vi "AlliGator Load HDF5 FLI Dataset Information.vi"(8 "Error In":errorcluster, 11 "File Path":path) -> (0 "error out":errorcluster, 1 "Data Description":string, 2 "Metadata":string, 3 "FLI Data File Information":T1, 4 "elapsed (relative) seconds":dbl)   [LabVIEW 2021, in "AlliGator HDF5.lvlib"]
doc: "Loads HDF5 FLI dataset information."
uses:
  AlliGator HDF5.lvlib
  AlliGator FLI Data File Information.ctl
  Phasor/Phasor Fluorescence Lifetime Parameters v3.ctl
  AlliGator FLI Dataset Type.ctl
  AlliGator HDF5 FLI File Loading Information v0.2.ctl
  Phasor/Fluorescence Lifetime Parameters.ctl
  AlliGator HDF5 FLI File Loading Information v0.6.ctl
  SwissSPAD/SwissSPAD Live_Image ROI Information.ctl
  AlliGator Image Binning Options.ctl
  Phasor/Phasor Fluorescence Lifetime Parameters v2.ctl
  <vilib>/addons/h5labview2/base/lib_path.vi
  <vilib>/addons/h5labview2/base/H5Equery.vi
  <vilib>/Utility/error.llb/Error Cluster From Error Code.vi
  AlliGator Load Single HDF5 Gate Image v 0.2b.vi
  AlliGator Load Single HDF5 Gate Image v 0.3b.vi
  AlliGator Load Single Gate Image from HDF5 v 0.6b.vi
  <vilib>/addons/h5labview2/base/hid_t.ctl
  <vilib>/addons/h5labview2/dataset/H5Dread.llb/H5Dread.xnode
  <vilib>/ErrorRing/Error Ring.xnode
  <vilib>/addons/h5labview2/file/H5F.lvlib
  <vilib>/addons/h5labview2/group/H5G.lvlib
  Time/Time.lvlib
  Phasor/Phasor.lvlib
  SwissSPAD/SwissSPAD Live.lvlib
  AlliGator Source Image.lvlib
  AlliGator Files.lvlib
  Variant/Variant.lvlib
panel:
  # "see the AlliGator License on the block diagram (Ctrl+E or Window:Show Block Diagram)"
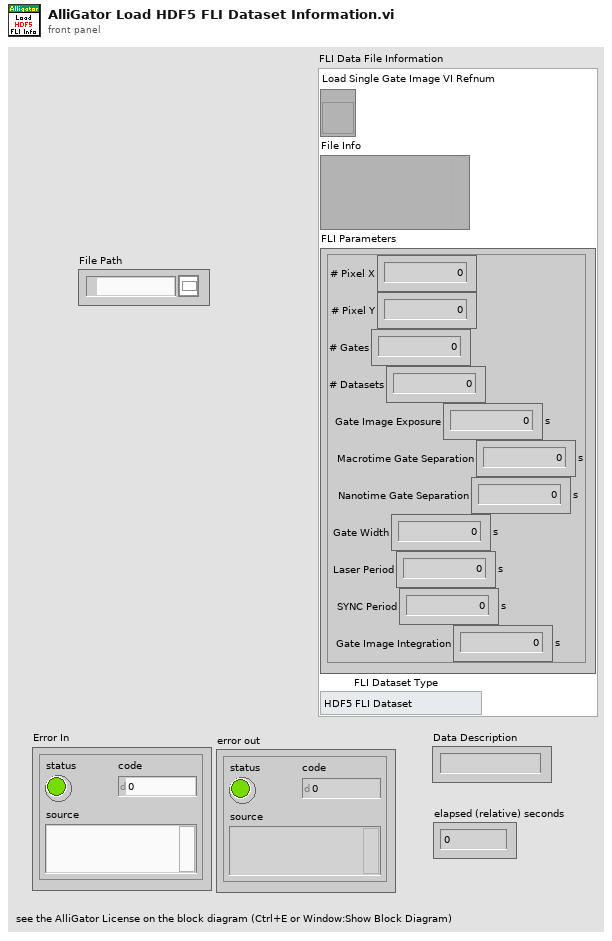
[diagram p1: front panel]
types:
  T1 = typedef "AlliGator HDF5.lvlib/AlliGator FLI Data File Information.ctl" = cluster{"Load Single Gate Image VI Refnum":refnum<vi>, "File Info":variant, "FLI Parameters":T2, "FLI Dataset Type":T3}
  T2 = typedef "Phasor.lvlib/Phasor Fluorescence Lifetime Parameters v3.ctl" = cluster{"# Pixel X":i32, "# Pixel Y":i32, "# Gates":i32, "# Datasets":i32, "Gate Image Exposure":dbl[unit], "Macrotime Gate Separation":dbl[unit], "Nanotime Gate Separation":dbl[unit], "Gate Width":dbl[unit], "Laser Period":dbl[unit], "SYNC Period":dbl[unit], "Gate Image Integration":dbl[unit]}
  T3 = typedef "AlliGator Files.lvlib/AlliGator FLI Dataset Type.ctl" = enum16{"HDF5 FLI Dataset", "Gate Image Folder", ".sdt FLI Dataset (Becker & Hickl)", ".ptu FLI Dataset (PicoQuant)", "SS1 FLI Dataset", "SS2 FLI Dataset", "I/m/phi Dataset", ".bin FLI Dataset (PicoQuant Binned)", ".bin FLI Dataset (Piccolo Binned)"}
  T4 = typedef "Phasor.lvlib/Fluorescence Lifetime Parameters.ctl" = cluster{"# Pixel X":i32, "# Pixel Y":i32, "# Gates":i32, "# Datasets":i32, "Exposure/Gate":dbl[unit], "Macrotime Gate Separation":dbl[unit], "Nanotime Gate Separation":dbl[unit], "Gate Duration":dbl[unit], "Laser Period":dbl[unit]}
  T5 = typedef "AlliGator HDF5.lvlib/AlliGator HDF5 FLI File Loading Information v0.2.ctl" = cluster{"HDF5 File Path":path}
  T6 = typedef "AlliGator HDF5.lvlib/AlliGator HDF5 FLI File Loading Information v0.6.ctl" = cluster{"HDF5 File Path":path, "Data Type":string, "# Datasets in Series":i32, "Dataset ID in Series":i32, "Channel Names":string[]}
  T7 = typedef "AlliGator Source Image.lvlib/AlliGator Image Binning Options.ctl" = cluster{"Use Image Binning":bool, "X Bin":i32, "Y Bin":i32}
  T8 = typedef "SwissSPAD Live.lvlib/SwissSPAD Live_Image ROI Information.ctl" = cluster{"Save ROI Only":bool, "Left":u16, "Top":u16, "Right":u16, "Bottom":u16, "Use Current ROI":bool}
  T9 = typedef "Phasor.lvlib/Phasor Fluorescence Lifetime Parameters v2.ctl" = cluster{"# Pixel X":i32, "# Pixel Y":i32, "# Gates":i32, "# Datasets":i32, "Exposure/Gate":dbl[unit], "Macrotime Gate Separation":dbl[unit], "Nanotime Gate Separation":dbl[unit], "Gate Duration":dbl[unit], "Laser Period":dbl[unit], "SYNC Period":dbl[unit]}
  T10 = typedef "hid_t.ctl" = i64
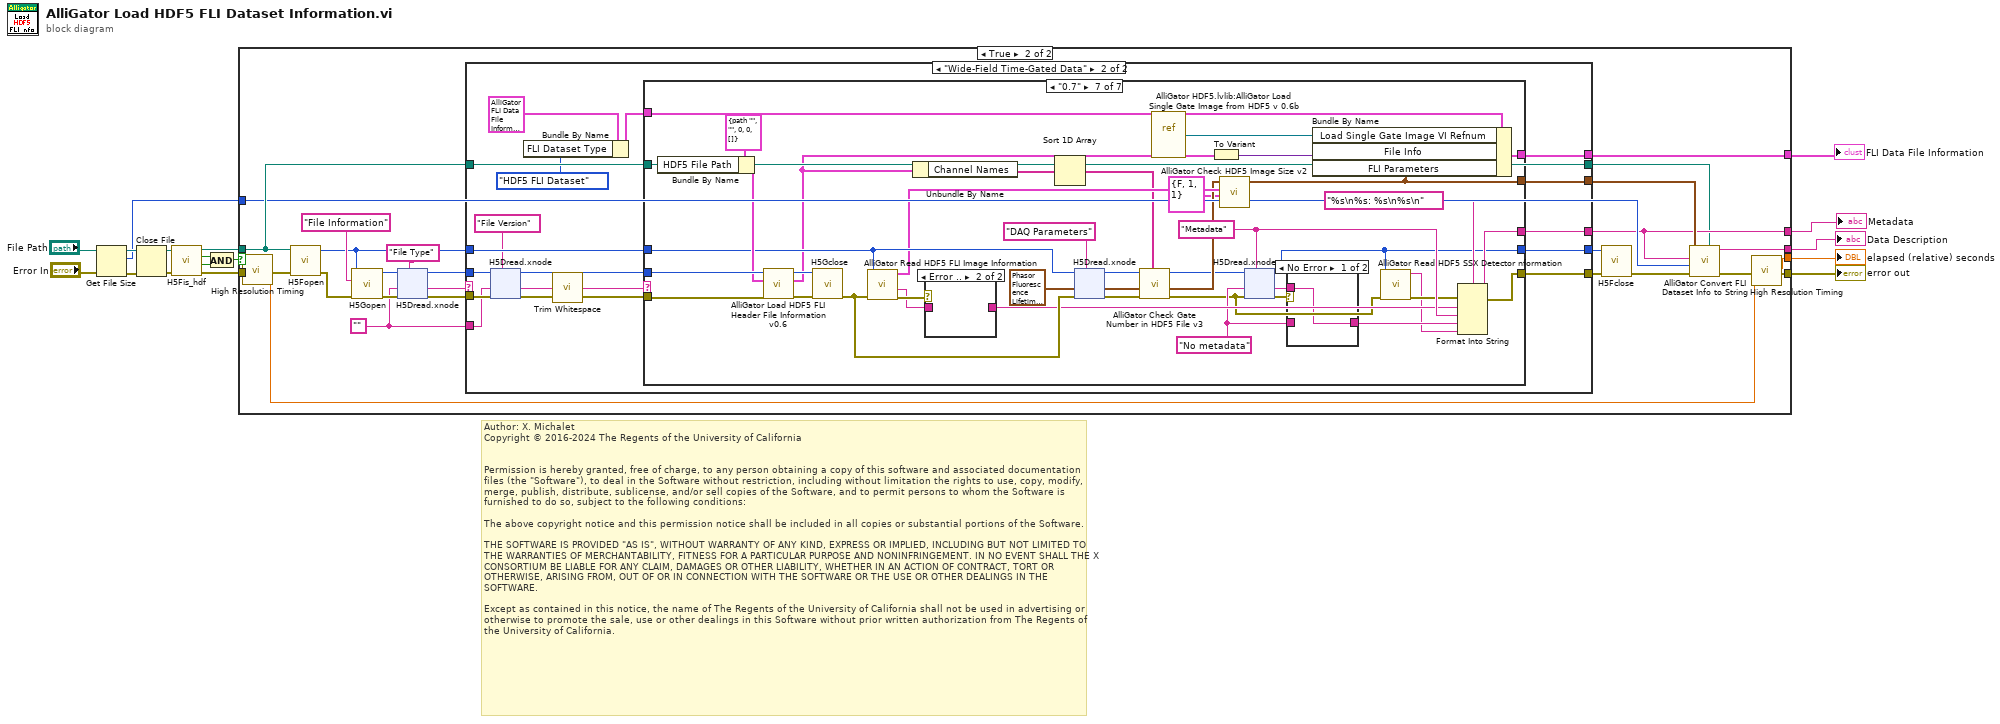
[diagram p0: block diagram]
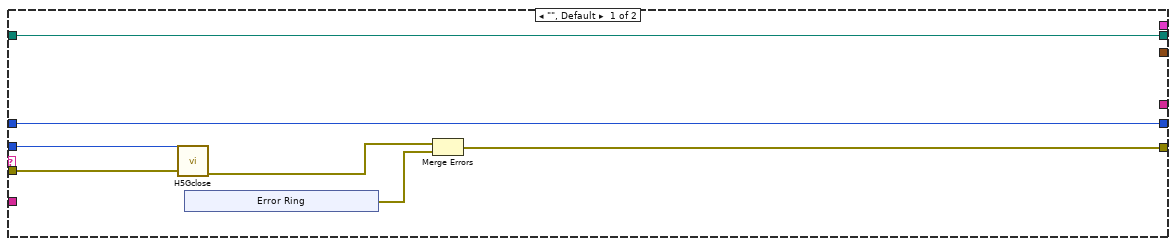
[diagram p3: hidden frame]
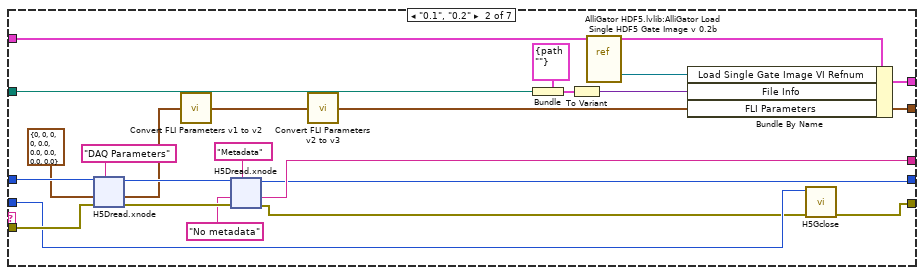
[diagram p5: hidden frame]
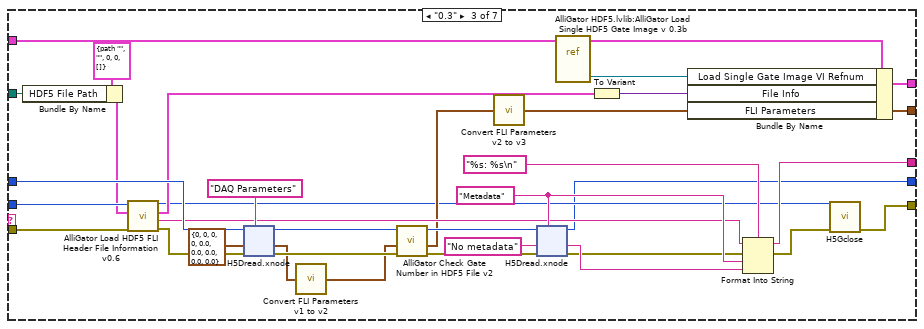
[diagram p6: hidden frame]
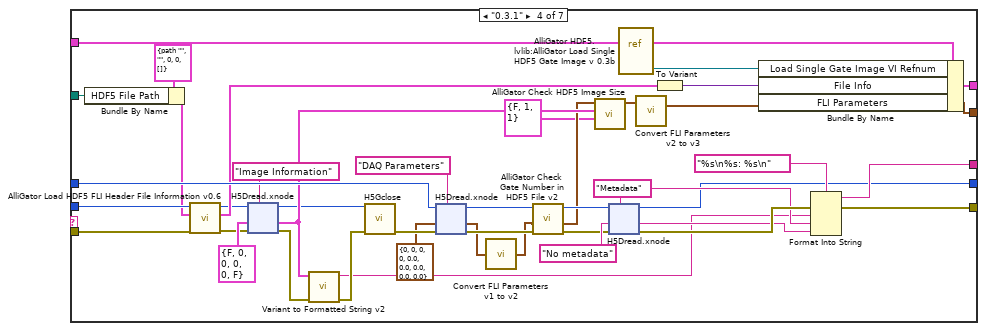
[diagram p7: hidden frame]
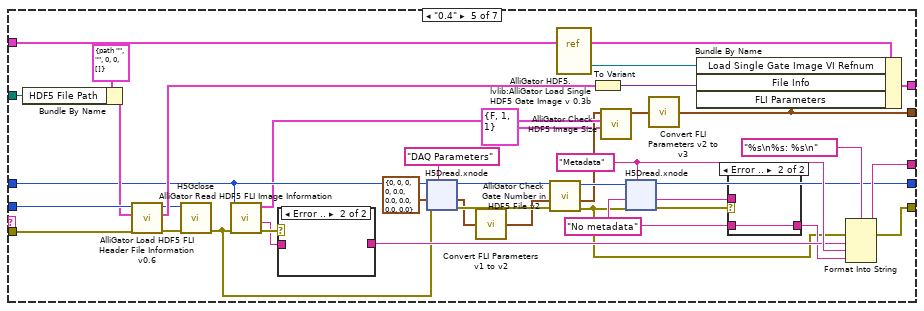
[diagram p8: hidden frame]
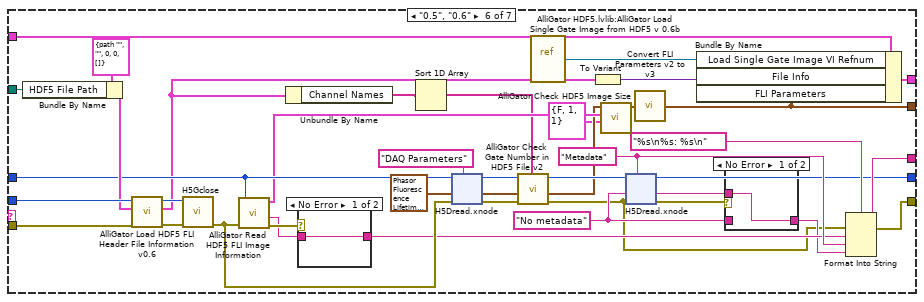
[diagram p11: hidden frame]
diagram:
  # "Author: X. Michalet\nCopyright © 2016-2024 The Regents of the University of California\n \n\nPermission is hereby granted, free of charge, to any person obtaining a copy of this software and associated documentation files (the \"Software\"), to deal in the Software without restriction, including without limitation the rights to use, copy, modify, merge, publish, distribute, sublicense, and/or sell copies of the Software, and to permit persons to whom the Software is furnished to do so, subject to the following conditions:\n\nThe above copyright notice and this permission notice shall be included in all copies or substantial portions of the Software.\n\nTHE SOFTWARE IS PROVIDED \"AS IS\", WITHOUT WARRANTY OF ANY KIND, EXPRESS OR IMPLIED, INCLUDING BUT NOT LIMITED TO THE WARRANTIES OF MERCHANTABILITY, FITNESS FOR A PARTICULAR PURPOSE AND NONINFRINGEMENT. IN NO EVENT SHALL THE X CONSORTIUM BE LIABLE FOR ANY CLAIM, DAMAGES OR OTHER LIABILITY, WHETHER IN AN ACTION OF CONTRACT, TORT OR OTHERWISE, ARISING FROM, OUT OF OR IN CONNECTION WITH THE SOFTWARE OR THE USE OR OTHER DEALINGS IN THE SOFTWARE.\n\nExcept as contained in this notice, the name of The Regents of the University of California shall not be used in advertising or otherwise to promote the sale, use or other dealings in this Software without prior written authorization from The Regents of the University of California."
  n1 = Get File Size(file="File Path", error in="Error In") -> (refnum out=w8:refnum<file>, size (in bytes)=w2:i64, 0:w9:errorcluster)
  n2 = Close File(refnum=w8, error in=w9) -> (path=w7:path, error out=w6:errorcluster)
  n3 = call <vilib>:"H5Fis_hdf.vi"("error in (no error)"=w6, "path in"=w7) -> ("error out"=w13:errorcluster, "valid?"=w16:bool, "exists?"=w17:bool, "path out"=w14:path)  [unwired: 6 in]
  n4 = And(x=w17, y=w16) -> (x .and. y?=w15:bool)
  n5 = case shown="True" w15 {
    tunnel: w14 -> [_ w27]
    tunnel: w13 -> [w18 w44]
    tunnel: [w18 w39] -> w12
    tunnel: [_ w37] -> w5
    tunnel: [_ w21] -> w4
    tunnel: [_ w26] -> w3
    tunnel: w2 -> [_ w23]
    tunnel: [_ w20] -> w1
    frame False {
    }
    frame True {
      w28 = ""
      n6 = call "High Resolution Timing.vi"("Error In"=w44) -> ("elapsed (relative) seconds"=w38:dbl, "Error Out"=w40:errorcluster)  [unwired: 16 in, 1 out]
      n7 = call <vilib>:"H5Fopen.vi"("error in (no error)"=w40, "path"=w27) -> ("error out"=w36:errorcluster, "ref out"=w31:T10)  [unwired: 8 in]
      n8 = call <vilib>:"H5Gopen.vi"("error in (no error)"=w36, "name"="File Information" ("dataset name (this)"), "ref in"=w31) -> ("error out"=w34:errorcluster, "group out"=w33:T10)  [unwired: 7 in]
      n9 = xnode "H5Dread.xnode"("dataset name (this)"="File Type", "error in (no error)"=w34, "default"=w28, "ref in"=w33) -> ("error out"=w30:errorcluster, "data"=w43:string, "ref out"=w29:T10)  [unwired: 2 in, 1 out]
      n10 = case shown="\"Wide-Field Time-Gated Data\"" w43 {
        tunnel: [w66 w88] -> w42
        tunnel: [w61 w74] -> w41
        tunnel: w31 -> [w66 w87]
        tunnel: w30 -> [w65 w85]
        tunnel: w28 -> [_ w84]
        tunnel: w29 -> [w64 w83]
        tunnel: [_ w81] -> w21
        tunnel: w27 -> [w62 w75]
        tunnel: [_ w79] -> w26
        tunnel: [_ w76] -> w22
        tunnel: [w62 w75] -> w19
        frame "", Default {
          n11 = call <vilib>:"H5Gclose.vi"("error in (no error)"=w65, "group in"=w64) -> ("error out"=w63:errorcluster)  [unwired: 9 in]
          n12 = xnode "Error Ring"() -> ("error out"=w60:errorcluster)
          n13 = Merge Errors(w63, w60) -> (w61:errorcluster)
        }
        frame "Wide-Field Time-Gated Data" {
          n14 = xnode "H5Dread.xnode"("dataset name (this)"="File Version", "error in (no error)"=w85, "default"=w84, "ref in"=w83) -> ("error out"=w78:errorcluster, "data"=w82:string, "ref out"=w77:T10)  [unwired: 2 in, 1 out]
          n15 = Bundle By Name(cluster=T1 {"Load Single Gate Image VI Refnum"=refnum, "File Info"=variant, "FLI Parameters"={"# Pixel X"=0, "# Pixel Y"=0, "# Gates"=0, "# Datasets"=0, "Gate Image Exposure"=0.0, "Macrotime Gate Separation"=0.0, "Nanotime Gate Separation"=0.0, "Gate Width"=0.0, "Laser Period"=0.0, "SYNC Period"=0.0, "Gate Image Integration"=0.0}, "FLI Dataset Type"=enum."HDF5 FLI Dataset"} ("FLI Data File Information"), "FLI Dataset Type"=AlliGator_FLI_Dataset_Type."HDF5 FLI Dataset") -> (w73:T1)
          n16 = call <vilib>:"Trim Whitespace.vi"("string"=w82) -> ("trimmed string"=w71:string)  [unwired: 1 in]
          n17 = case shown="\"0.7\"" w71 {
            tunnel: w87 -> [w105 w127 w191 w262 w325 w400 w476]
            tunnel: w78 -> [w104 w128 w183 w254 w339 w413 w487]
            tunnel: [w105 w107 w159 w240 w328 w403 w459] -> w88
            tunnel: [w104 w111 w165 w226 w336 w410 w484] -> w74
            tunnel: [_ w121 w180 w252 w337 w411 w485] -> w81
            tunnel: w73 -> [_ w120 w187 w258 w343 w416 w490]
            tunnel: w75 -> [_ w119 w181 w253 w338 w412 w486]
            tunnel: [_ w117 w185 w256 w341 w415 w489] -> w79
            tunnel: w77 -> [_ w112 w184 w255 w340 w414 w488]
            tunnel: [_ w108 w161 w222 w308 w382 w460] -> w76
            frame "", Default {
            }
            frame "0.1", "0.2" {
              n18 = xnode "H5Dread.xnode"("dataset name (this)"="DAQ Parameters", "error in (no error)"=w128, "default"=T4 {"# Pixel X"=0, "# Pixel Y"=0, "# Gates"=0, "# Datasets"=0, "Exposure/Gate"=0.0, "Macrotime Gate Separation"=0.0, "Nanotime Gate Separation"=0.0, "Gate Duration"=0.0, "Laser Period"=0.0} ("FLI Parameters"), "ref in"=w127) -> ("error out"=w125:errorcluster, "data"=w116:T4, "ref out"=w124:i64)  [unwired: 2 in, 1 out]
              n19 = call "Convert FLI Parameters v1 to v2.vi"("FLI Parameters"=w116) -> ("FLI Parameters v2"=w109:T9)  [unwired: 8 in]
              n20 = xnode "H5Dread.xnode"("dataset name (this)"="Metadata" ("dataset name"), "error in (no error)"=w125, "default"="No metadata" ("type name (default)"), "ref in"=w124) -> ("error out"=w106:errorcluster, "data"=w121:string, "ref out"=w107:T10)  [unwired: 2 in, 1 out]
              n21 = call "Convert FLI Parameters v2 to v3.vi"("FLI Parameters v2"=w109) -> ("FLI Parameters v3"=w108:T2)
              n22 = Bundle(cluster=T5 {"HDF5 File Path"=path ""} ("output cluster"), "HDF5 File Path"=w119) -> (w114:T5)
              n23 = To Variant(anything=w114) -> (Variant=w115:variant)
              n24 = vi-ref "AlliGator HDF5.lvlib:AlliGator Load Single HDF5 Gate Image v 0.2b.vi"() -> (w118:refnum<vi>)
              n25 = Bundle By Name(cluster=w120, "Load Single Gate Image VI Refnum"=w118, "File Info"=w115, "FLI Parameters"=w108) -> (w117:T1)
              n26 = call <vilib>:"H5Gclose.vi"("error in (no error)"=w106, "group in"=w112) -> ("error out"=w111:errorcluster)  [unwired: 9 in]
            }
            frame "0.3" {
              w179 = "Metadata" ("dataset name")
              n27 = Bundle By Name(cluster=T6 {"HDF5 File Path"=path "", "Data Type"="", "# Datasets in Series"=0, "Dataset ID in Series"=0, "Channel Names"=[]} ("output cluster"), "HDF5 File Path"=w181) -> (w172:T6)
              n28 = call "AlliGator Load HDF5 FLI Header File Information v0.6.vi"("error in (no error)"=w183, "HDF5 FLI File Loading Information"=w172, "ref in"=w184) -> ("error out"=w182:errorcluster, "File Information String"=w174:string, "HDF5 FLI File Loading Information out"=w171:T6, "ref out"=w166:T10)  [unwired: 5 in]
              n29 = xnode "H5Dread.xnode"("dataset name (this)"="DAQ Parameters", "error in (no error)"=w182, "default"=T4 {"# Pixel X"=0, "# Pixel Y"=0, "# Gates"=0, "# Datasets"=0, "Exposure/Gate"=0.0, "Macrotime Gate Separation"=0.0, "Nanotime Gate Separation"=0.0, "Gate Duration"=0.0, "Laser Period"=0.0} ("FLI Parameters"), "ref in"=w191) -> ("error out"=w189:errorcluster, "data"=w163:T4, "ref out"=w188:T10)  [unwired: 2 in, 1 out]
              n30 = call "Convert FLI Parameters v1 to v2.vi"("FLI Parameters"=w163) -> ("FLI Parameters v2"=w162:T9)  [unwired: 8 in]
              n31 = call "AlliGator Check Gate Number in HDF5 File v2.vi"("error in (no error)"=w189, "FLI Parameters"=w162, "ref in"=w188) -> ("error out"=w170:errorcluster, "FLI Parameters"=w168:T9, "ref"=w169:T10)  [unwired: 4 in, 2 out]
              n32 = call "Convert FLI Parameters v2 to v3.vi"("FLI Parameters v2"=w168) -> ("FLI Parameters v3"=w161:T2)
              n33 = xnode "H5Dread.xnode"("dataset name (this)"=w179, "error in (no error)"=w170, "default"="No metadata" ("type name (default)"), "ref in"=w169) -> ("error out"=w160:errorcluster, "data"=w177:string, "ref out"=w159:T10)  [unwired: 2 in, 1 out]
              n34 = vi-ref "AlliGator HDF5.lvlib:AlliGator Load Single HDF5 Gate Image v 0.3b.vi"() -> (w186:refnum<vi>)
              n35 = To Variant(anything=w171) -> (Variant=w176:variant)
              n36 = Bundle By Name(cluster=w187, "Load Single Gate Image VI Refnum"=w186, "File Info"=w176, "FLI Parameters"=w161) -> (w185:T1)
              n37 = Format Into String(format string="%s: %s\n", initial string=w174, error in=w160, w179, w177) -> (resulting string=w180:string, error out=w167:errorcluster)
              n38 = call <vilib>:"H5Gclose.vi"("error in (no error)"=w167, "group in"=w166) -> ("error out"=w165:errorcluster)  [unwired: 9 in]
            }
            frame "0.3.1" {
              w243 = "Metadata" ("dataset name")
              n39 = Bundle By Name(cluster=T6 {"HDF5 File Path"=path "", "Data Type"="", "# Datasets in Series"=0, "Dataset ID in Series"=0, "Channel Names"=[]} ("output cluster"), "HDF5 File Path"=w253) -> (w246:T6)
              n40 = call "AlliGator Load HDF5 FLI Header File Information v0.6.vi"("error in (no error)"=w254, "HDF5 FLI File Loading Information"=w246, "ref in"=w255) -> ("error out"=w235:errorcluster, "HDF5 FLI File Loading Information out"=w245:T6, "ref out"=w236:T10)  [unwired: 5 in, 1 out]
              n41 = xnode "H5Dread.xnode"("dataset name (this)"="Image Information" ("name"), "error in (no error)"=w235, "default"=T8 {"Save ROI Only"=FALSE, "Left"=0, "Top"=0, "Right"=0, "Bottom"=0, "Use Current ROI"=FALSE} ("Image Information"), "ref in"=w236) -> ("error out"=w237:errorcluster, "data"=w233:T8, "ref out"=w230:T10)  [unwired: 2 in, 1 out]
              n42 = call "Variant to Formatted String v2.vi"("error in (no error)"=w237, "Anything"=w233) -> ("error out"=w229:errorcluster, "String"=w227:string)  [unwired: 8 in]
              n43 = call <vilib>:"H5Gclose.vi"("error in (no error)"=w229, "group in"=w230) -> ("error out"=w228:errorcluster)  [unwired: 9 in]
              n44 = xnode "H5Dread.xnode"("dataset name (this)"="DAQ Parameters", "error in (no error)"=w228, "default"=T4 {"# Pixel X"=0, "# Pixel Y"=0, "# Gates"=0, "# Datasets"=0, "Exposure/Gate"=0.0, "Macrotime Gate Separation"=0.0, "Nanotime Gate Separation"=0.0, "Gate Duration"=0.0, "Laser Period"=0.0} ("FLI Parameters"), "ref in"=w262) -> ("error out"=w260:errorcluster, "data"=w224:T4, "ref out"=w259:T10)  [unwired: 2 in, 1 out]
              n45 = call "Convert FLI Parameters v1 to v2.vi"("FLI Parameters"=w224) -> ("FLI Parameters v2"=w223:T9)  [unwired: 8 in]
              n46 = call "AlliGator Check Gate Number in HDF5 File v2.vi"("error in (no error)"=w260, "FLI Parameters"=w223, "ref in"=w259) -> ("error out"=w242:errorcluster, "FLI Parameters"=w232:T9, "ref"=w241:T10)  [unwired: 4 in, 2 out]
              n47 = call "AlliGator Check HDF5 Image Size.vi"("Image Binning Options"=T7 {"Use Image Binning"=FALSE, "X Bin"=1, "Y Bin"=1}, "Image ROI Information"=w233, "FLI Parameters in"=w232) -> ("FLI Parameters out"=w234:T9)  [unwired: 8 in]
              n48 = xnode "H5Dread.xnode"("dataset name (this)"=w243, "error in (no error)"=w242, "default"="No metadata" ("type name (default)"), "ref in"=w241) -> ("error out"=w251:errorcluster, "data"=w244:string, "ref out"=w240:T10)  [unwired: 2 in, 1 out]
              n49 = vi-ref "AlliGator HDF5.lvlib:AlliGator Load Single HDF5 Gate Image v 0.3b.vi"() -> (w257:refnum<vi>)
              n50 = call "Convert FLI Parameters v2 to v3.vi"("FLI Parameters v2"=w234) -> ("FLI Parameters v3"=w222:T2)
              n51 = To Variant(anything=w245) -> (Variant=w249:variant)
              n52 = Bundle By Name(cluster=w258, "Load Single Gate Image VI Refnum"=w257, "File Info"=w249, "FLI Parameters"=w222) -> (w256:T1)
              n53 = Format Into String(format string="%s\n%s: %s\n", error in=w251, w227, w243, w244) -> (resulting string=w252:string, error out=w226:errorcluster)  [unwired: 1 in]
            }
            frame "0.4" {
              w311 = "No metadata" ("type name (default)")
              w330 = "Metadata" ("dataset name")
              n54 = Bundle By Name(cluster=T6 {"HDF5 File Path"=path "", "Data Type"="", "# Datasets in Series"=0, "Dataset ID in Series"=0, "Channel Names"=[]} ("output cluster"), "HDF5 File Path"=w338) -> (w332:T6)
              n55 = call "AlliGator Load HDF5 FLI Header File Information v0.6.vi"("error in (no error)"=w339, "HDF5 FLI File Loading Information"=w332, "ref in"=w340) -> ("error out"=w326:errorcluster, "HDF5 FLI File Loading Information out"=w331:T6, "ref out"=w327:T10)  [unwired: 5 in, 1 out]
              n56 = call <vilib>:"H5Gclose.vi"("error in (no error)"=w326, "group in"=w327) -> ("error out"=w314:errorcluster)  [unwired: 9 in]
              n57 = call "AlliGator Read HDF5 FLI Image Information.vi"("error in (no error)"=w314, "ref in"=w325) -> ("error out"=w317:errorcluster, "Image Information"=w316:string, "Image ROI Information"=w324:T8)  [unwired: 6 in, 1 out]
              n58 = case shown="Error .." w317 {
                tunnel: [w379 _] -> w315
                tunnel: w316 -> [w379 _]
                frame No Error {
                }
                frame Error {
                }
              }
              n59 = xnode "H5Dread.xnode"("dataset name (this)"="DAQ Parameters", "error in (no error)"=w314, "default"=T4 {"# Pixel X"=0, "# Pixel Y"=0, "# Gates"=0, "# Datasets"=0, "Exposure/Gate"=0.0, "Macrotime Gate Separation"=0.0, "Nanotime Gate Separation"=0.0, "Gate Duration"=0.0, "Laser Period"=0.0} ("FLI Parameters"), "ref in"=w325) -> ("error out"=w345:errorcluster, "data"=w319:T4, "ref out"=w344:T10)  [unwired: 2 in, 1 out]
              n60 = call "Convert FLI Parameters v1 to v2.vi"("FLI Parameters"=w319) -> ("FLI Parameters v2"=w318:T9)  [unwired: 8 in]
              n61 = call "AlliGator Check Gate Number in HDF5 File v2.vi"("error in (no error)"=w345, "FLI Parameters"=w318, "ref in"=w344) -> ("error out"=w309:errorcluster, "FLI Parameters"=w323:T9, "ref"=w329:T10)  [unwired: 4 in, 2 out]
              n62 = vi-ref "AlliGator HDF5.lvlib:AlliGator Load Single HDF5 Gate Image v 0.3b.vi"() -> (w342:refnum<vi>)
              n63 = To Variant(anything=w331) -> (Variant=w335:variant)
              n64 = call "AlliGator Check HDF5 Image Size.vi"("Image Binning Options"=T7 {"Use Image Binning"=FALSE, "X Bin"=1, "Y Bin"=1}, "Image ROI Information"=w324, "FLI Parameters in"=w323) -> ("FLI Parameters out"=w322:T9)  [unwired: 8 in]
              n65 = xnode "H5Dread.xnode"("dataset name (this)"=w330, "error in (no error)"=w309, "default"=w311, "ref in"=w329) -> ("error out"=w312:errorcluster, "data"=w313:string, "ref out"=w328:T10)  [unwired: 2 in, 1 out]
              n66 = call "Convert FLI Parameters v2 to v3.vi"("FLI Parameters v2"=w322) -> ("FLI Parameters v3"=w308:T2)
              n67 = Bundle By Name(cluster=w343, "Load Single Gate Image VI Refnum"=w342, "File Info"=w335, "FLI Parameters"=w308) -> (w341:T1)
              n68 = case shown="Error .." w312 {
                tunnel: [w377 w378] -> w310
                tunnel: w311 -> [_ w378]
                tunnel: w313 -> [w377 _]
                frame No Error {
                }
                frame Error {
                }
              }
              n69 = Format Into String(format string="%s\n%s: %s\n", error in=w309, w315, w330, w310) -> (resulting string=w337:string, error out=w336:errorcluster)  [unwired: 1 in]
            }
            frame "0.5", "0.6" {
              w388 = "No metadata" ("type name (default)")
              w405 = "Metadata" ("dataset name")
              n70 = Bundle By Name(cluster=T6 {"HDF5 File Path"=path "", "Data Type"="", "# Datasets in Series"=0, "Dataset ID in Series"=0, "Channel Names"=[]} ("output cluster"), "HDF5 File Path"=w412) -> (w406:T6)
              n71 = call "AlliGator Load HDF5 FLI Header File Information v0.6.vi"("error in (no error)"=w413, "HDF5 FLI File Loading Information"=w406, "ref in"=w414) -> ("error out"=w401:errorcluster, "HDF5 FLI File Loading Information out"=w383:T6, "ref out"=w402:T10)  [unwired: 5 in, 1 out]
              n72 = call <vilib>:"H5Gclose.vi"("error in (no error)"=w401, "group in"=w402) -> ("error out"=w392:errorcluster)  [unwired: 9 in]
              n73 = call "AlliGator Read HDF5 FLI Image Information.vi"("error in (no error)"=w392, "ref in"=w400) -> ("error out"=w393:errorcluster, "Image Information"=w391:string, "Image ROI Information"=w399:T8)  [unwired: 6 in, 1 out]
              n74 = Unbundle By Name(w383) -> ("Channel Names"=w381:string[])
              n75 = case shown="No Error" w393 {
                tunnel: [w452 _] -> w390
                tunnel: w391 -> [w452 _]
                frame No Error {
                }
                frame Error {
                }
              }
              n76 = Sort 1D Array(array=w381) -> (sorted array=w380:string[])
              n77 = xnode "H5Dread.xnode"("dataset name (this)"="DAQ Parameters", "error in (no error)"=w392, "default"=T9 {"# Pixel X"=0, "# Pixel Y"=0, "# Gates"=0, "# Datasets"=0, "Exposure/Gate"=0.0, "Macrotime Gate Separation"=0.0, "Nanotime Gate Separation"=0.0, "Gate Duration"=0.0, "Laser Period"=0.0, "SYNC Period"=0.0} ("Swiss SPAD File Information"), "ref in"=w400) -> ("error out"=w418:errorcluster, "data"=w394:T9, "ref out"=w417:i64)  [unwired: 2 in, 1 out]
              n78 = call "AlliGator Check Gate Number in HDF5 File v2.vi"("Gate Names"=w380, "error in (no error)"=w418, "FLI Parameters"=w394, "ref in"=w417) -> ("error out"=w385:errorcluster, "FLI Parameters"=w398:T9, "ref"=w404:T10)  [unwired: 3 in, 2 out]
              n79 = vi-ref "AlliGator HDF5.lvlib:AlliGator Load Single Gate Image from HDF5 v 0.6b.vi"() -> (w384:refnum<vi>)
              n80 = To Variant(anything=w383) -> (Variant=w409:variant)
              n81 = call "AlliGator Check HDF5 Image Size.vi"("Image Binning Options"=T7 {"Use Image Binning"=FALSE, "X Bin"=1, "Y Bin"=1}, "Image ROI Information"=w399, "FLI Parameters in"=w398) -> ("FLI Parameters out"=w397:T9)  [unwired: 8 in]
              n82 = xnode "H5Dread.xnode"("dataset name (this)"=w405, "error in (no error)"=w385, "default"=w388, "ref in"=w404) -> ("error out"=w389:errorcluster, "data"=w386:string, "ref out"=w403:T10)  [unwired: 2 in, 1 out]
              n83 = call "Convert FLI Parameters v2 to v3.vi"("FLI Parameters v2"=w397) -> ("FLI Parameters v3"=w382:T2)
              n84 = Bundle By Name(cluster=w416, "Load Single Gate Image VI Refnum"=w384, "File Info"=w409, "FLI Parameters"=w382) -> (w415:T1)
              n85 = case shown="No Error" w389 {
                tunnel: [w450 w451] -> w387
                tunnel: w388 -> [_ w451]
                tunnel: w386 -> [w450 _]
                frame No Error {
                }
                frame Error {
                }
              }
              n86 = Format Into String(format string="%s\n%s: %s\n", error in=w385, w390, w405, w387) -> (resulting string=w411:string, error out=w410:errorcluster)  [unwired: 1 in]
            }
            frame "0.7" {
              w465 = "No metadata" ("type name (default)")
              w479 = "Metadata" ("dataset name")
              n87 = Bundle By Name(cluster=T6 {"HDF5 File Path"=path "", "Data Type"="", "# Datasets in Series"=0, "Dataset ID in Series"=0, "Channel Names"=[]} ("output cluster"), "HDF5 File Path"=w486) -> (w480:T6)
              n88 = call "AlliGator Load HDF5 FLI Header File Information v0.6.vi"("error in (no error)"=w487, "HDF5 FLI File Loading Information"=w480, "ref in"=w488) -> ("error out"=w477:errorcluster, "HDF5 FLI File Loading Information out"=w461:T6, "ref out"=w478:T10)  [unwired: 5 in, 1 out]
              n89 = call <vilib>:"H5Gclose.vi"("error in (no error)"=w477, "group in"=w478) -> ("error out"=w469:errorcluster)  [unwired: 9 in]
              n90 = call "AlliGator Read HDF5 FLI Image Information.vi"("error in (no error)"=w469, "ref in"=w476) -> ("error out"=w470:errorcluster, "Image Information"=w468:string, "Image ROI Information"=w475:T8)  [unwired: 6 in, 1 out]
              n91 = Unbundle By Name(w461) -> ("Channel Names"=w454:string[])
              n92 = case shown="Error .." w470 {
                tunnel: [w526 _] -> w467
                tunnel: w468 -> [w526 _]
                frame No Error {
                }
                frame Error {
                }
              }
              n93 = Sort 1D Array(array=w454) -> (sorted array=w453:string[])
              n94 = xnode "H5Dread.xnode"("dataset name (this)"="DAQ Parameters", "error in (no error)"=w469, "default"=T2 {"# Pixel X"=0, "# Pixel Y"=0, "# Gates"=0, "# Datasets"=0, "Gate Image Exposure"=0.0, "Macrotime Gate Separation"=0.0, "Nanotime Gate Separation"=0.0, "Gate Width"=0.0, "Laser Period"=0.0, "SYNC Period"=0.0, "Gate Image Integration"=0.0} ("Swiss SPAD File Information"), "ref in"=w476) -> ("error out"=w492:errorcluster, "data"=w471:T2, "ref out"=w491:T10)  [unwired: 2 in, 1 out]
              n95 = call "AlliGator Check Gate Number in HDF5 File v3.vi"("Gate Names"=w453, "error in (no error)"=w492, "FLI Parameters"=w471, "ref in"=w491) -> ("error out"=w458:errorcluster, "FLI Parameters"=w474:T2, "ref"=w455:T10)  [unwired: 3 in, 2 out]
              n96 = vi-ref "AlliGator HDF5.lvlib:AlliGator Load Single Gate Image from HDF5 v 0.6b.vi"() -> (w462:refnum<vi>)
              n97 = To Variant(anything=w461) -> (Variant=w483:variant)
              n98 = call "AlliGator Check HDF5 Image Size v2.vi"("Image Binning Options"=T7 {"Use Image Binning"=FALSE, "X Bin"=1, "Y Bin"=1}, "Image ROI Information"=w475, "FLI Parameters in"=w474) -> ("FLI Parameters out"=w460:T2)  [unwired: 8 in]
              n99 = xnode "H5Dread.xnode"("dataset name (this)"=w479, "error in (no error)"=w458, "default"=w465, "ref in"=w455) -> ("error out"=w466:errorcluster, "data"=w463:string, "ref out"=w459:T10)  [unwired: 2 in, 1 out]
              n100 = case shown="No Error" w466 {
                tunnel: [w524 w525] -> w464
                tunnel: w465 -> [_ w525]
                tunnel: w463 -> [w524 _]
                frame No Error {
                }
                frame Error {
                }
              }
              n101 = Bundle By Name(cluster=w490, "Load Single Gate Image VI Refnum"=w462, "File Info"=w483, "FLI Parameters"=w460) -> (w489:T1)
              n102 = call "AlliGator Read HDF5 SSX Detector nformation.vi"("error in (no error)"=w458, "ref in"=w459) -> ("error out"=w457:errorcluster, "SwissSPAD Detector Information"=w456:string)  [unwired: 8 in]
              n103 = Format Into String(format string="%s\n%s: %s\n%s\n", error in=w457, w467, w479, w464, w456) -> (resulting string=w485:string, error out=w484:errorcluster)  [unwired: 1 in]
            }
          }
        }
      }
      n104 = call <vilib>:"H5Fclose.vi"("error in (no error)"=w41, "ref"=w42) -> ("error out"=w25:errorcluster)  [unwired: 9 in]
      n105 = call "AlliGator Convert FLI Dataset Info to String.vi"("File Path"=w19, "error in (no error)"=w25, "size"=w23, "Metadata"=w21, "FLI Parameters"=w22) -> ("Error Out"=w24:errorcluster, "Data Description"=w20:string)  [unwired: 5 in]
      n106 = call "High Resolution Timing.vi"("relative seconds (NaN)"=w38, "Error In"=w24) -> ("elapsed (relative) seconds"=w37:dbl, "Error Out"=w39:errorcluster)  [unwired: 15 in, 1 out]
    }
  }
  "error out" <- w12
  "elapsed (relative) seconds" <- w5
  "Metadata" <- w4
  "FLI Data File Information" <- w3
  "Data Description" <- w1
